vi "Calculator.vi"() -> ()   [LabVIEW 2020]
panel:
  in  "Ring":u16(ring) items=["Add", "Sub", "Mult", "Div"]
  out "y":dbl
  in  "x2":dbl
  in  "x1":dbl
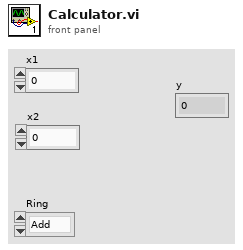
[diagram p1: front panel]
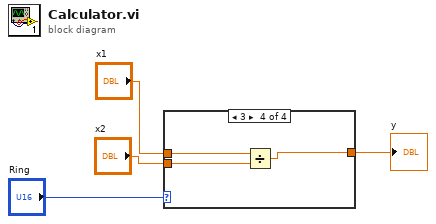
[diagram p0: block diagram]
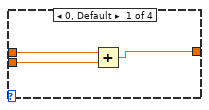
[diagram p2: hidden frame]
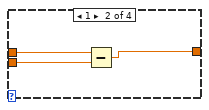
[diagram p3: hidden frame]
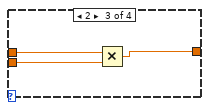
[diagram p4: hidden frame]
diagram:
  n1 = case shown="3" "Ring" {
    tunnel: "x1" -> [w7 w10 w13 w16]
    tunnel: "x2" -> [w6 w9 w12 w15]
    tunnel: [w5 w8 w11 w14] -> w2
    frame 0, Default {
      n2 = Add(x=w7, y=w6) -> (x+y=w5:dbl)
    }
    frame 1 {
      n3 = Subtract(x=w10, y=w9) -> (x-y=w8:dbl)
    }
    frame 2 {
      n4 = Multiply(x=w13, y=w12) -> (x*y=w11:dbl)
    }
    frame 3 {
      n5 = Divide(x=w16, y=w15) -> (x/y=w14:dbl)
    }
  }
  "y" <- w2
